vi "Main For Loop.vi"(11 "80 32 Bit Words out":bool[][](array[boolean])) -> (0 "D Out":bool[](array[boolean]), 1 "C out":bool[](array[boolean]), 2 "B Out":bool[](array[boolean]), 3 "A Out":bool[](array[boolean]), 4 "E Out":bool[](array[boolean]))   [LabVIEW 2013]
panel:
  out "K 4":bool[](array[boolean])
  out "K 3":bool[](array[boolean])
  out "K 2":bool[](array[boolean])
  out "K":bool[](array[boolean])
  out "F":bool[](array[boolean])
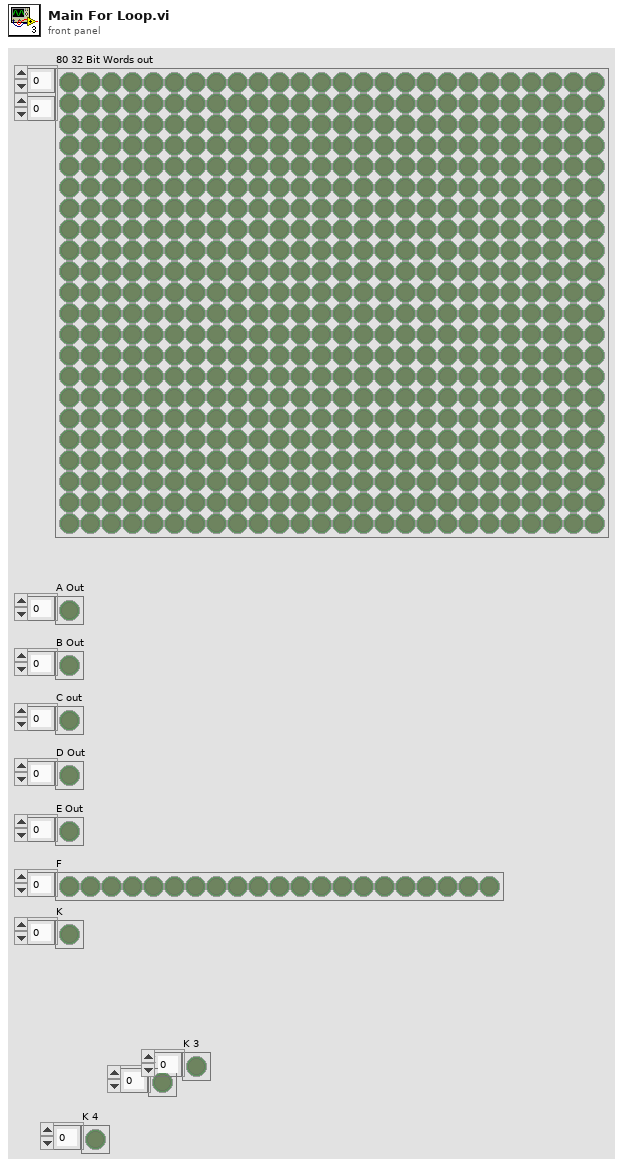
[diagram p1: front panel]
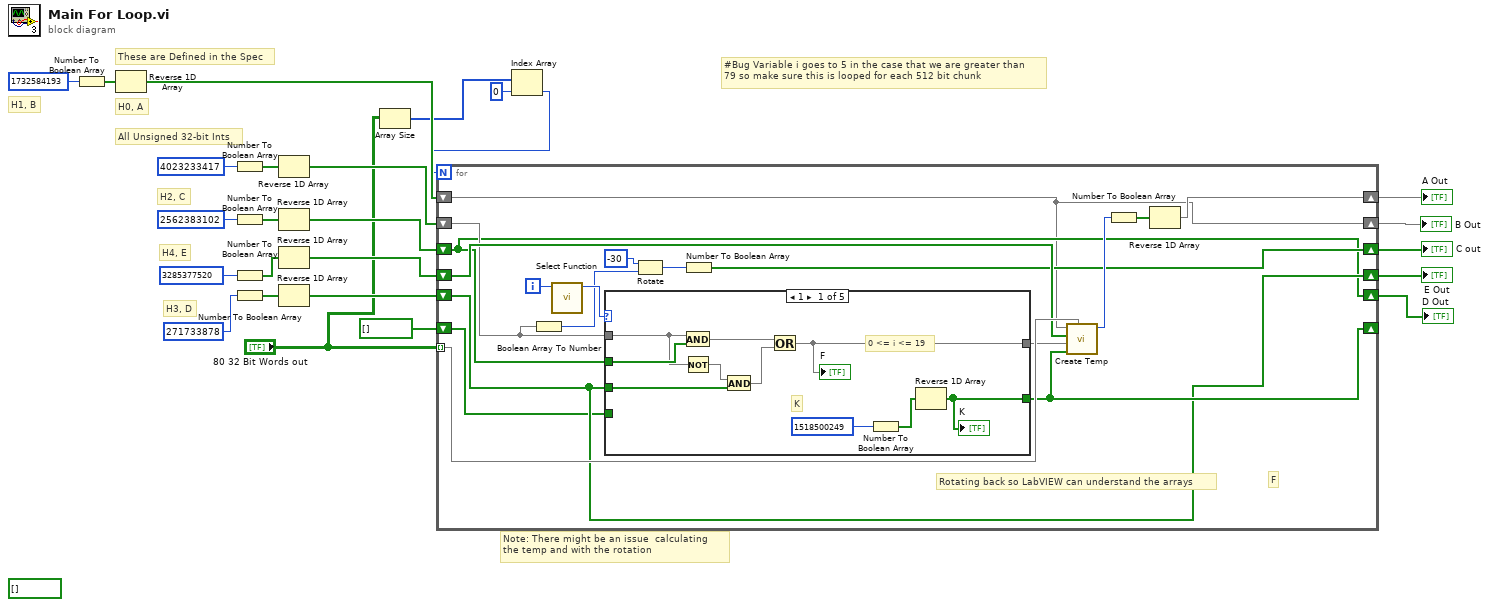
[diagram p0: block diagram]
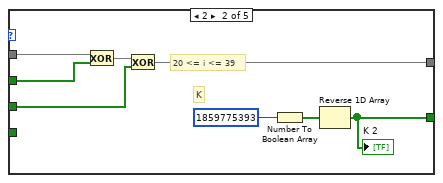
[diagram p2: hidden frame]
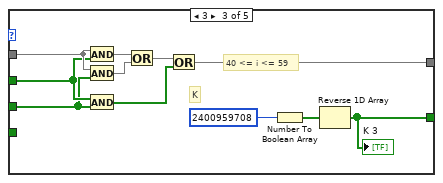
[diagram p3: hidden frame]
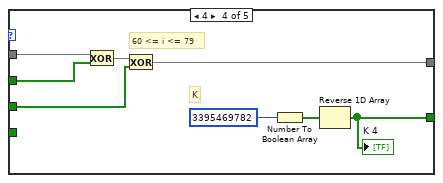
[diagram p4: hidden frame]
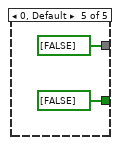
[diagram p5: hidden frame]
diagram:
  (unwired) bool[] []
  # "#Bug Variable i goes to 5 in the case that we are greater than \n79 so make sure this is looped for each 512 bit chunk"
  # "Note: There might be an issue  calculating \nthe temp and with the rotation"
  # "These are Defined in the Spec"
  # "All Unsigned 32-bit Ints"
  # "H0, A"
  # "H4, E"
  # "H3, D"
  # "H2, C"
  # "H1, B"
  n1 = Number To Boolean Array(number=u32 1732584193) -> (Boolean array=w20:bool[])
  n2 = Reverse 1D Array(array=w20) -> (reversed array=w11:bool[])
  n3 = Number To Boolean Array(number=u32 4023233417) -> (Boolean array=w19:bool[])
  n4 = Number To Boolean Array(number=u32 2562383102) -> (Boolean array=w18:bool[])
  n5 = Number To Boolean Array(number=u32 3285377520) -> (Boolean array=w16:bool[])
  n6 = Number To Boolean Array(number=u32 271733878) -> (Boolean array=w17:bool[])
  n7 = Reverse 1D Array(array=w19) -> (reversed array=w14:bool[])
  n8 = Reverse 1D Array(array=w18) -> (reversed array=w15:bool[])
  n9 = Reverse 1D Array(array=w16) -> (reversed array=w12:bool[])
  n10 = Reverse 1D Array(array=w17) -> (reversed array=w13:bool[])
  n11 = Array Size(array="80 32 Bit Words out") -> (size(s)=w8:i32[])
  n12 = Index Array(array=w8, index=0) -> (element=w6:i32)
  n13 = for {
    N: w6 -> [_]
    shift-right: [w28] -> w1
    shift-left: w14 -> [w34]
    shift-right: [w29] -> w4
    shift-left: w13 -> [w35]
    shift-right: [w30] -> w3
    shift-left: w15 -> [w29]
    shift-right: [w35] -> w2
    shift-left: w12 -> [w40]
    shift-right: [w36] -> w5
    shift-left: w11 -> [w28]
    shift-right: [w39] -> _
    shift-left: bool[] [] -> [w26]
    tunnel: "80 32 Bit Words out" -> [w41] mode=indexing
    i -> [w42]
    # "Rotating back so LabVIEW can understand the arrays"
    # "F"
    n14 = Boolean Array To Number(Boolean array=w34) -> (number=w33:u32)
    n15 = call "Select Function.vi"("Numeric"=w42) -> ("result"=w43:i32)  [unwired: 10 in]
    n16 = case shown="1" w43 {
      tunnel: w29 -> [w53 w57 w68 w76 _]
      tunnel: w34 -> [w52 w58 w69 w77 _]
      tunnel: w35 -> [w51 w55 w67 w74 _]
      tunnel: [w45 w59 w70 w78 bool[] [FALSE]] -> w39
      tunnel: w26 -> [_ _ _ _ _]
      tunnel: [w44 w54 w62 w73 bool[] [FALSE]] -> w27
      frame 1 {
        # "0 <= i <= 19"
        # "K"
        n17 = And(x=w52, y=w53) -> (x .and. y?=w49:bool[])
        n18 = Not(x=w52) -> (.not. x?=w50:bool[])
        n19 = And(x=w50, y=w51) -> (x .and. y?=w48:bool[])
        n20 = Or(x=w49, y=w48) -> (x .or. y?=w44:bool[])
        "F" <- w44
        n21 = Number To Boolean Array(number=u32 1518500249) -> (Boolean array=w46:bool[])
        n22 = Reverse 1D Array(array=w46) -> (reversed array=w45:bool[])
        "K" <- w45
      }
      frame 2 {
        # "20 <= i <= 39"
        # "K"
        n23 = Exclusive Or(1:w57, 2:w58) -> (0:w56:bool[])
        n24 = Exclusive Or(1:w55, 2:w56) -> (0:w54:bool[])
        n25 = Number To Boolean Array(number=u32 1859775393) -> (Boolean array=w60:bool[])
        n26 = Reverse 1D Array(array=w60) -> (reversed array=w59:bool[])
        "K 2" <- w59
      }
      frame 3 {
        # "K"
        # "40 <= i <= 59"
        n27 = And(x=w69, y=w68) -> (x .and. y?=w66:bool[])
        n28 = And(x=w69, y=w67) -> (x .and. y?=w65:bool[])
        n29 = And(x=w68, y=w67) -> (x .and. y?=w63:bool[])
        n30 = Or(x=w66, y=w65) -> (x .or. y?=w64:bool[])
        n31 = Or(x=w64, y=w63) -> (x .or. y?=w62:bool[])
        n32 = Number To Boolean Array(number=u32 2400959708) -> (Boolean array=w71:bool[])
        n33 = Reverse 1D Array(array=w71) -> (reversed array=w70:bool[])
        "K 3" <- w70
      }
      frame 4 {
        # "K"
        # "60 <= i <= 79"
        n34 = Exclusive Or(1:w76, 2:w77) -> (0:w75:bool[])
        n35 = Exclusive Or(1:w74, 2:w75) -> (0:w73:bool[])
        n36 = Number To Boolean Array(number=u32 3395469782) -> (Boolean array=w79:bool[])
        n37 = Reverse 1D Array(array=w79) -> (reversed array=w78:bool[])
        "K 4" <- w78
      }
      frame 0, Default {
      }
    }
    n38 = Rotate(1:w33, 2:i16 -30 ("y")) -> (0:w31:u32)
    n39 = Number To Boolean Array(number=w31) -> (Boolean array=w30:bool[])
    n40 = call "Create Temp.vi"("Word In"=w41, "K"=w39, "F"=w27, "E"=w40, "A"=w28) -> ("unsigned 32bit integer"=w38:u32)  [unwired: 6 in]
    n41 = Number To Boolean Array(number=w38) -> (Boolean array=w37:bool[])
    n42 = Reverse 1D Array(array=w37) -> (reversed array=w36:bool[])
  }
  "A Out" <- w5
  "D Out" <- w4
  "C out" <- w3
  "E Out" <- w2
  "B Out" <- w1
